vi "Destroy.vi"(8 "error in (no error)":errorcluster, 11 "Graph In":refnum<class "Graph.lvclass">) -> (0 "error out":errorcluster, 3 "Graph Out":refnum<class "Graph.lvclass">)   [LabVIEW 2017, in "Front Panel Publisher.lvlib" / "Graph.lvclass"]
uses:
  Graph.lvclass
  Control_class/Control.lvclass
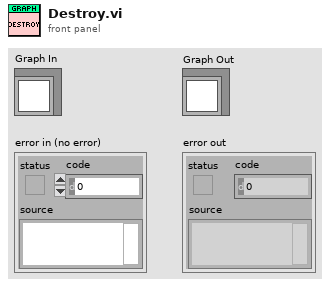
[diagram p1: front panel]
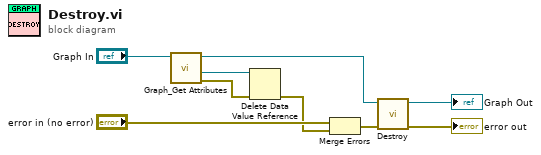
[diagram p0: block diagram]
diagram:
  n1 = call "Graph_Get Attributes.vi"("reference in"="Graph In") -> ("error out"=w2:errorcluster, "Graph DVR"=w3:refnum<data-value>, "reference out"=w4:refnum<class "Graph.lvclass">)  [unwired: 7 in, 1 out]
  n2 = Delete Data Value Reference(data value reference=w3, error in=w2) -> (error out=w1:errorcluster)  [unwired: 1 out]
  n3 = Merge Errors("error in (no error)", w1) -> (w7:errorcluster)
  n4 = call-parent "Destroy.vi"("error in (no error)"=w7, "Control In"=w4) -> ("error out"=→"error out":errorcluster, "Control Out"=→"Graph Out":refnum<class "Graph.lvclass">)  [unwired: 8 in]
